vi "Find Autonomous Play Files.vi"(0 "Application Directory":path, 1 "User Path Input":string, 2 "Do not include file\nsuffix":bool) -> (3 "FileName\nFilepath\nArray":cluster{string, string}[](array[cluster]), 4 "Application Directory":path, 5 "Filepath Array":string[](array[string]), 6 "filename array":string[](array[string]))   [LabVIEW 2015]
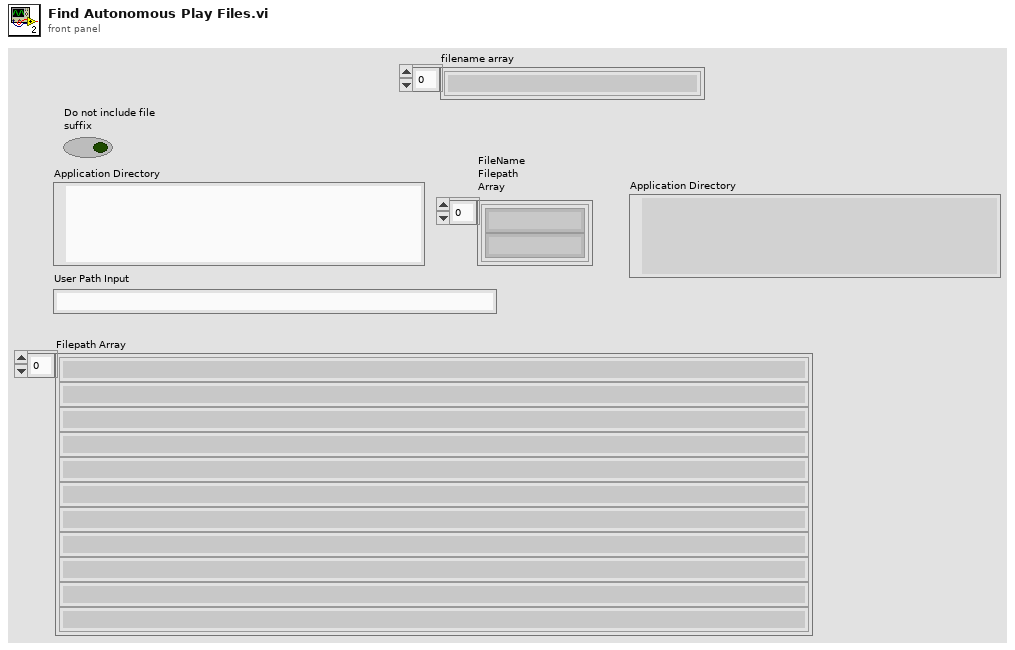
[diagram p1: front panel]
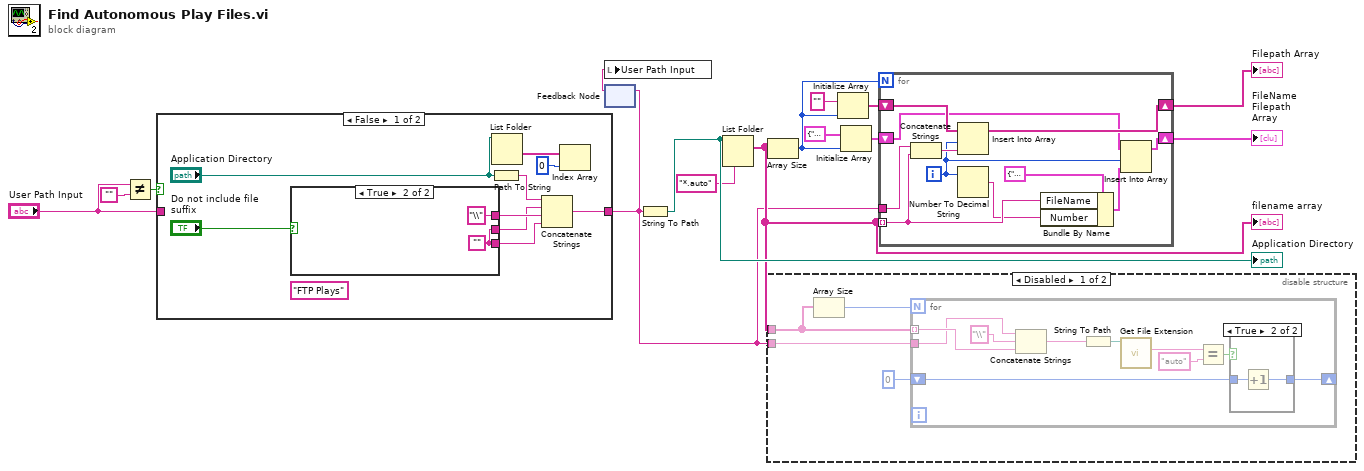
[diagram p0: block diagram]
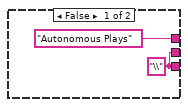
[diagram p4: hidden frame]
diagram:
  n1 = Not Equal?(x="User Path Input", y="") -> (x != y?=w3:bool)
  n2 = case shown="False" w3 {
    tunnel: [w18 w29] -> w2
    tunnel: "User Path Input" -> [_ w29]
    frame False {
      (unwired) "FTP Plays" ("string")
      n3 = case shown="True" "Do not include file\nsuffix" {
        tunnel: ["Autonomous Plays" ("string") "\\" ("string")] -> w21
        tunnel: [w25 w28] -> w20
        tunnel: [w25 w28] -> w16
        frame False {
          w25 = "\\" ("string")
        }
        frame True {
          w28 = ""
        }
      }
      n4 = Path To String(path="Application Directory") -> (string=w19:string)
      n5 = List Folder(path="Application Directory") -> (folder names=w23:string[])  [unwired: 3 in, 3 out]
      n6 = Concatenate Strings(w19, w20, w21, w16) -> (w18:string)
      n7 = Index Array(array=w23, index=0) -> ()  [unwired: 1 out]
    }
    frame True {
    }
  }
  n8 = feedback-in #1(w2) -> ()
  n9 = feedback #1() -> (w1:string)  [unwired: 1 in]
  n10 = local write "User Path Input"(w1) -> ()
  n11 = String To Path(string=w2) -> (path=w8:path)
  "Application Directory" <- w8
  n12 = List Folder(path=w8, pattern="*.auto") -> (filenames=w5:string[])  [unwired: 2 in, 3 out]
  "filename array" <- w5
  n13 = Array Size(array=w5) -> (size(s)=w10:i32)
  n14 = disable-structure shown="Disabled" {
    disable-tunnel: w5 -> [w32 _]
    disable-tunnel: w2 -> [w31 _]
    frame Disabled {
      n15 = Array Size(array=w32) -> (size(s)=w33:i32)
      n16 = for {
        N: w33 -> [_]
        tunnel: w32 -> [w40] mode=indexing
        tunnel: w31 -> [w39]
        shift-right: [w36] -> _
        shift-left: 0 -> [w34]
        n17 = Concatenate Strings(w39, "\\", w40) -> (w42:string)
        n18 = String To Path(string=w42) -> (path=w43:path)
        n19 = call <vilib>:"Get File Extension.vi"("file"=w43) -> ("lowercase file extension"=w38:string)  [unwired: 6 in, 4 out]
        n20 = Equal?(x=w38, y="auto") -> (x = y?=w35:bool)
        n21 = case shown="True" w35 {
          tunnel: [w44 w46] -> w36
          tunnel: w34 -> [w44 w45]
          frame False {
          }
          frame True {
            n22 = Increment(x=w45) -> (x+1=w46:i32)
          }
        }
      }
    }
    frame Enabled {
    }
  }
  n23 = Initialize Array("", w10) -> (w14:string[])
  n24 = Initialize Array(cluster{string, string} {"", ""}, w10) -> (w12:cluster{string, string}[])
  n25 = for {
    N: w10 -> [_]
    tunnel: w5 -> [w54] mode=indexing
    tunnel: w2 -> [w57]
    shift-right: [w53] -> w15
    shift-left: w14 -> [w52]
    shift-right: [w49] -> w9
    shift-left: w12 -> [w51]
    i -> [w47]
    n26 = Concatenate Strings(w57, w54) -> (w55:string)
    n27 = Insert Into Array(array=w52, index=w47, new element=w55) -> (w53:string[])
    n28 = Number To Decimal String(number=w47) -> (decimal integer string=w48:string)  [unwired: 1 in]
    n29 = Bundle By Name(cluster=cluster{"FileName":string, "Number":string} {"FileName"="", "Number"=""} ("input cluster"), "FileName"=w54, "Number"=w48) -> (w50:cluster{"FileName":string, "Number":string})
    n30 = Insert Into Array(array=w51, index=w47, new element=w50) -> (w49:cluster{string, string}[])
  }
  "Filepath Array" <- w15
  "FileName\nFilepath\nArray" <- w9
